vi "DSF.Engine.Framework.Error Handler.vi"(8 "error in (no error)":errorcluster, 11 "Framework in":refnum<class "DSF.Engine.Framework.lvclass">) -> (0 "error out":errorcluster, 3 "Framework out":refnum<class "DSF.Engine.Framework.lvclass">)   [LabVIEW 2017, in "Data Sharing Framework Engine.lvlib" / "DSF.Engine.Framework.lvclass"]
uses:
  DSF.Engine.Framework.lvclass
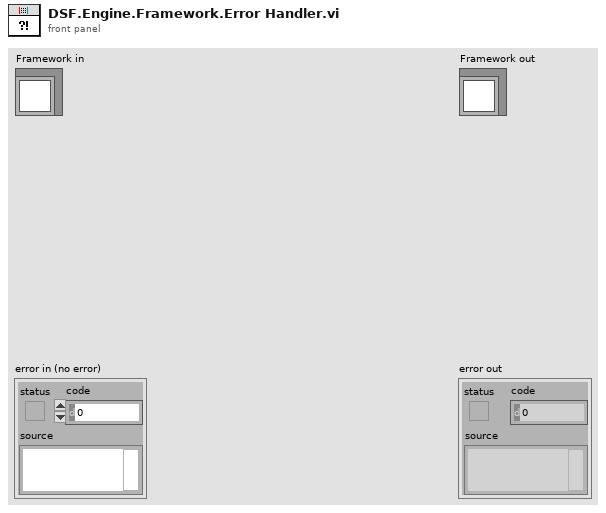
[diagram p1: front panel]
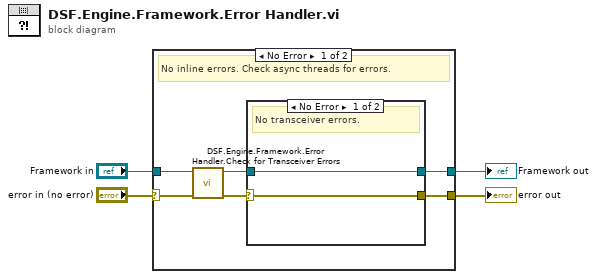
[diagram p0: block diagram]
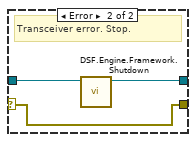
[diagram p2: hidden frame]
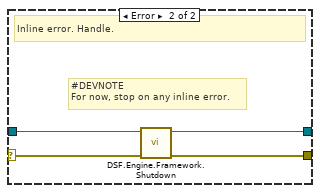
[diagram p3: hidden frame]
diagram:
  n1 = case shown="No Error" "error in (no error)" {
    selector: "error in (no error)" -> [w9 w19]
    tunnel: "Framework in" -> [w10 w18]
    tunnel: [w6 w17] -> w3
    tunnel: [w5 w16] -> w2
    frame No Error {
      # "No inline errors. Check async threads for errors."
      n2 = call "DSF.Engine.Framework.Error Handler.Check for Transceiver Errors.vi"("error in (no error)"=w9, "Framework in"=w10) -> ("error out"=w8:errorcluster, "Framework out"=w7:refnum<class "DSF.Engine.Framework.lvclass">)  [unwired: 8 in]
      n3 = case shown="No Error" w8 {
        selector: w8 -> [w11 w13]
        tunnel: w7 -> [w12 w15]
        tunnel: [w12 w14] -> w6
        tunnel: [w11 w13] -> w5
        frame No Error {
          # "No transceiver errors."
        }
        frame Error {
          # "Transceiver error. Stop."
          n4 = call "DSF.Engine.Framework.Shutdown.vi"("Framework in"=w15) -> ("Framework out"=w14:refnum<class "DSF.Engine.Framework.lvclass">)  [unwired: 9 in, 1 out]
        }
      }
    }
    frame Error {
      # "#DEVNOTE\nFor now, stop on any inline error."
      # "Inline error. Handle."
      n5 = call "DSF.Engine.Framework.Shutdown.vi"("error in (no error)"=w19, "Framework in"=w18) -> ("error out"=w16:errorcluster, "Framework out"=w17:refnum<class "DSF.Engine.Framework.lvclass">)  [unwired: 8 in]
    }
  }
  "error out" <- w2
  "Framework out" <- w3
